vi "IntensityGraph.vi"(8 "error in (no error)":errorcluster, 10 "GameRef":refnum<class "Game.lvclass">, 11 "Evaluator in":refnum<class "Evaluator.lvclass">) -> (0 "error out":errorcluster, 2 "Intensity Graph":dbl[][](graph), 3 "Evaluator out":refnum<class "Evaluator.lvclass">)   [LabVIEW 2023, in "Evaluator.lvclass"]
uses:
  Evaluator.lvclass
  Game_class/Game.lvclass
  Game_class/Game.lvclass/Game.ctl
  Game_class/Read FieldRef.vi
  Field_class/Field.lvclass
panel:
  in  "Threshold":i32=100
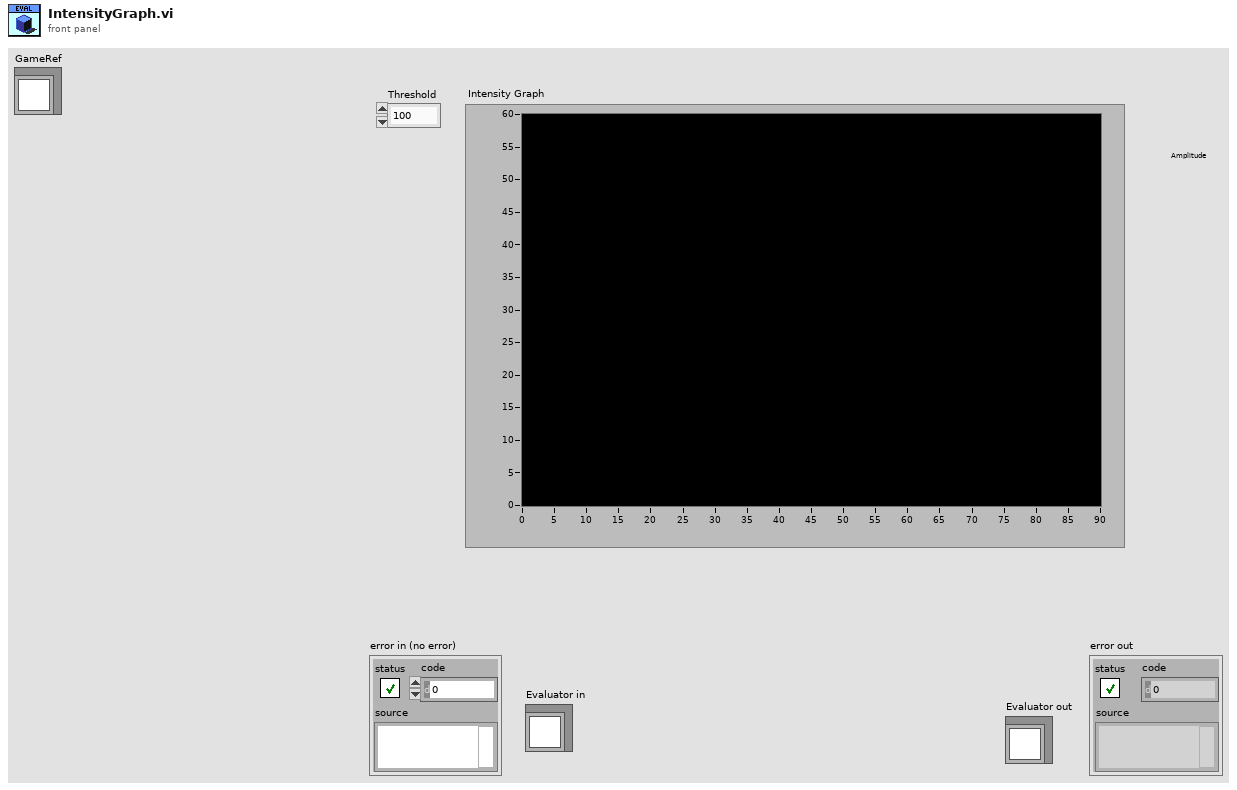
[diagram p1: front panel]
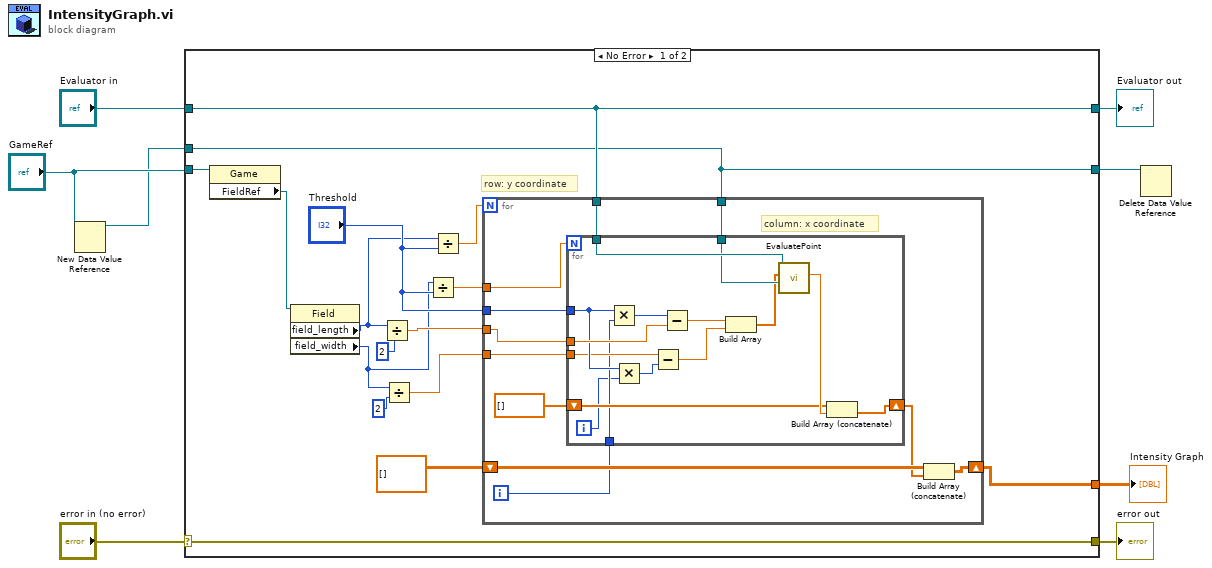
[diagram p0: block diagram]
diagram:
  n1 = New Data Value Reference(data value="GameRef") -> (data value reference=w2:refnum<data-value>)  [unwired: 1 in, 1 out]
  n2 = case shown="No Error" "error in (no error)" {
    selector: "error in (no error)" -> [w24 w53]
    tunnel: [w24 w53] -> w7
    tunnel: [w18 w52] -> w5
    tunnel: "Evaluator in" -> [w18 w52]
    tunnel: "GameRef" -> [w23 _]
    tunnel: [w19 _] -> w4
    tunnel: w2 -> [w9 w51]
    tunnel: [w9 w51] -> w1
    frame No Error {
      # "row: y coordinate"
      n3 = property class="Game"(reference=w23) -> ("FieldRef"=w22:refnum<class "Field.lvclass">)  [unwired: 1 in, 2 out]
      n4 = property class="Field"(reference=w22) -> ("field_length"=w12:i32, "field_width"=w15:i32)  [unwired: 1 in, 2 out]
      n5 = Divide(x=w12, y=2) -> (x/y=w16:dbl)
      n6 = Divide(x=w15, y=2) -> (x/y=w13:dbl)
      n7 = Divide(x=w15, y="Threshold") -> (x/y=w11:dbl)
      n8 = Divide(x=w12, y="Threshold") -> (x/y=w10:dbl)
      n9 = for {
        N: w10 -> [_]
        shift-right: [w34] -> w19
        shift-left: dbl[][] [] -> [w35]
        tunnel: w18 -> [w31]
        tunnel: w9 -> [w30]
        tunnel: "Threshold" -> [w29]
        tunnel: w16 -> [w28]
        tunnel: w13 -> [w27]
        tunnel: w11 -> [w25]
        i -> [w26]
        # "column: x coordinate"
        n10 = for {
          N: w25 -> [_]
          shift-right: [w50] -> w33
          shift-left: dbl[] [] -> [w48]
          tunnel: w31 -> [w47]
          tunnel: w30 -> [w46]
          tunnel: w29 -> [w43]
          tunnel: w28 -> [w44]
          tunnel: w27 -> [w42]
          tunnel: w26 -> [w37]
          i -> [w36]
          n11 = Multiply(x=w43, y=w37) -> (x*y=w45:i32)
          n12 = Multiply(x=w43, y=w36) -> (x*y=w41:i32)
          n13 = Subtract(x=w42, y=w41) -> (x-y=w38:dbl)
          n14 = Subtract(x=w45, y=w44) -> (x-y=w39:dbl)
          n15 = Build Array(w39, w38) -> (w40:dbl[])
          n16 = call-dynamic "EvaluatePoint.vi"("GameRef"=w46, "Point"=w40, "Evaluator in"=w47) -> ("Evaluation"=w49:dbl)  [unwired: 6 in, 2 out]
          n17 = Build Array (concatenate)(w48, w49) -> (w50:dbl[])
        }
        n18 = Build Array (concatenate)(w35, w33) -> (w34:dbl[][])
      }
    }
    frame Error {
    }
  }
  "error out" <- w7
  "Evaluator out" <- w5
  "Intensity Graph" <- w4
  n19 = Delete Data Value Reference(data value reference=w1) -> ()  [unwired: 1 in, 2 out]
